vi "Load Bar.vi"(8 "error in":errorcluster) -> (0 "error out":errorcluster)   [LabVIEW 2024, in "User Interface.lvlib"]
uses:
  User Interface.lvlib
  Support/General Type Defs/Global Data.vi
  Support/General Type Defs/General Type Definitions.lvlib
panel:
  out "Loadbar":dbl(slide) scale=0.0..100.0
  # "Looking for active sessions"
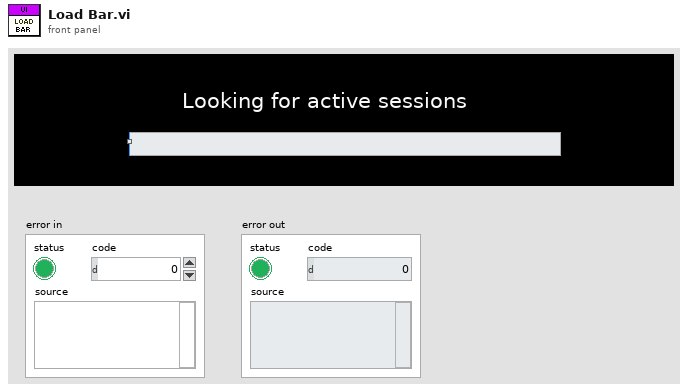
[diagram p1: front panel]
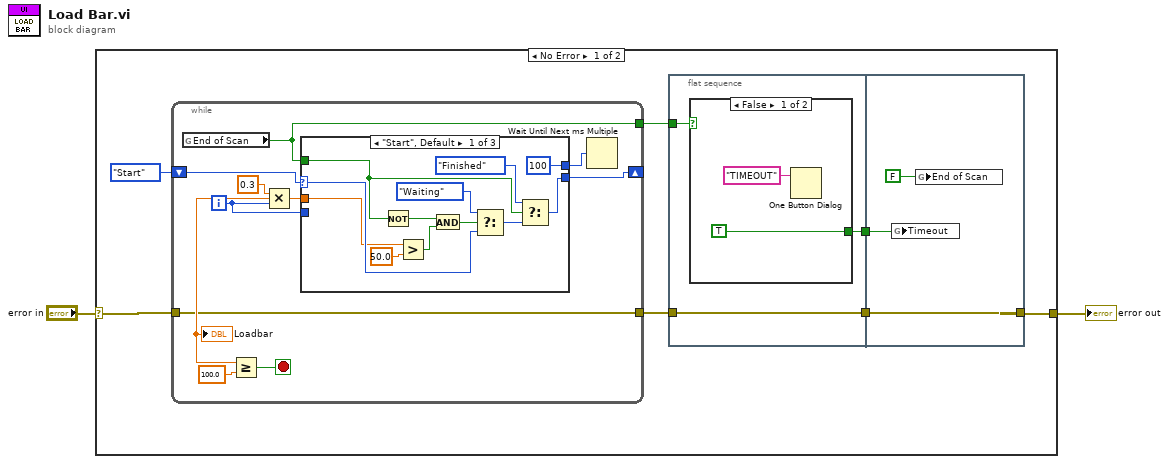
[diagram p0: block diagram]
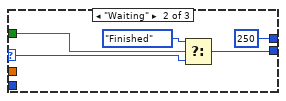
[diagram p3: hidden frame]
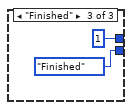
[diagram p4: hidden frame]
diagram:
  n1 = case shown="No Error" "error in" {
    selector: "error in" -> [w8 _]
    tunnel: [w6 _] -> w1
    frame No Error {
      n2 = while {
        shift-right: [w23] -> _
        shift-left: enum16{"Start", "Waiting", "Finished"}."Start" -> [w25]
        tunnel: w8 -> [w19]
        tunnel: [w19] -> w7
        tunnel: [w18] -> w4
        i -> [w24]
        stop <- w27 stop-if-true
        n3 = global read "Global Data.vi" "End of Scan"() -> (w18:bool)
        n4 = Multiply(x=0.3, y=w24) -> (x*y=w21:dbl)
        "Loadbar" <- w21
        n5 = Greater Or Equal?(x=w21, y=100.0) -> (x >= y?=w27:bool)
        n6 = case shown="\"Start\", Default" w25 {
          selector: w25 -> [w31 w40 _]
          tunnel: w24 -> [_ _ _]
          tunnel: w18 -> [w34 w42 _]
          tunnel: [w30 w43 enum16{"Start", "Waiting", "Finished"}."Finished"] -> w23
          tunnel: w21 -> [w29 _ _]
          tunnel: [u32 100 ("millisecond multiple") u32 250 ("millisecond multiple") u32 1 ("millisecond multiple")] -> w20
          frame "Start", Default {
            n7 = Not(x=w34) -> (.not. x?=w37:bool)
            n8 = Greater?(x=w29, y=50.0) -> (0:w38:bool)
            n9 = And(x=w37, y=w38) -> (x .and. y?=w36:bool)
            n10 = Select(t=enum16{"Start", "Waiting", "Finished"}."Waiting", s=w36, f=w31) -> (s? t:f=w35:enum16{"Start", "Waiting", "Finished"})
            n11 = Select(t=enum16{"Start", "Waiting", "Finished"}."Finished", s=w34, f=w35) -> (s? t:f=w30:enum16{"Start", "Waiting", "Finished"})
          }
          frame "Waiting" {
            n12 = Select(t=enum16{"Start", "Waiting", "Finished"}."Finished", s=w42, f=w40) -> (s? t:f=w43:enum16{"Start", "Waiting", "Finished"})
          }
          frame "Finished" {
          }
        }
        n13 = Wait Until Next ms Multiple(millisecond multiple=w20) -> ()  [unwired: 1 out]
      }
      n14 = flat-sequence {
        tunnel: w7 -> [w12]
        tunnel: [w12] -> w5
        tunnel: w4 -> [w11]
        tunnel: [w10] -> w3
        tunnel: [w17] -> w6
        tunnel: w5 -> [w17]
        tunnel: w3 -> [w15]
        frame #0 {
          n15 = case shown="False" w11 {
            tunnel: [TRUE ("End of Scan") _] -> w10
            frame False {
              n16 = One Button Dialog(message="TIMEOUT") -> ()  [unwired: 1 in, 1 out]
            }
            frame True {
            }
          }
        }
        frame #1 {
          n17 = global write "Global Data.vi" "Timeout"(w15) -> ()
          n18 = global write "Global Data.vi" "End of Scan"(FALSE ("End of Scan")) -> ()
        }
      }
    }
    frame Error {
    }
  }
  "error out" <- w1
